vi "taskPrototype.vi"(8 "error in (no error)":errorcluster, 10 "stopMechanism":refnum<class "ITaskStopMechanism.lvclass">, 11 "ITask in":refnum<class "ITask.lvclass">) -> (0 "error out":errorcluster, 3 "ITask out":refnum<class "ITask.lvclass">)   [LabVIEW 2023]
doc: "_____________________________________\nTLC Daemon 1.0.0.2\nCopyright (c) 2026 Andrea Cadei"
uses:
  ITask/ITask.lvclass
  ITaskStopMechanism/ITaskStopMechanism.lvclass
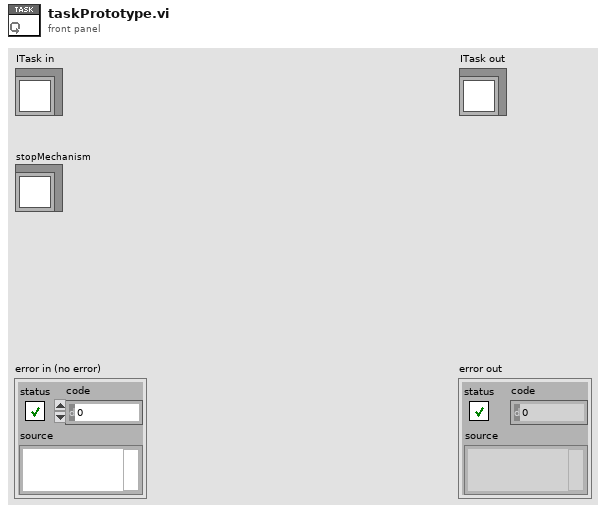
[diagram p1: front panel]
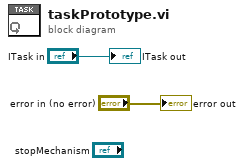
[diagram p0: block diagram]
diagram:
  "error out" <- "error in (no error)"
  "ITask out" <- "ITask in"
